vi "writePre.vi"(1 "input_data":u8[](array[numeric]) format="%.0x", 2 "address":u8, 3 "Channel":u8 max=5 step=1, 4 "order":u8[](array[numeric])=[238, 0, 13, 0, 1, 160, 0, 0, 169, 255, 252, 255, 255] format="%.0x") -> (0 "out":u8[](array[numeric]) format="%.0x")   [LabVIEW 2011]
panel:
  out "输出数组":u8[](array[numeric]) format="%.0x"
  out "size":u8
  # "channel"
  # "芯片地址"
  # "写入字节数"
  # "读写控制"
  # "字节数"
  # "写入地址"
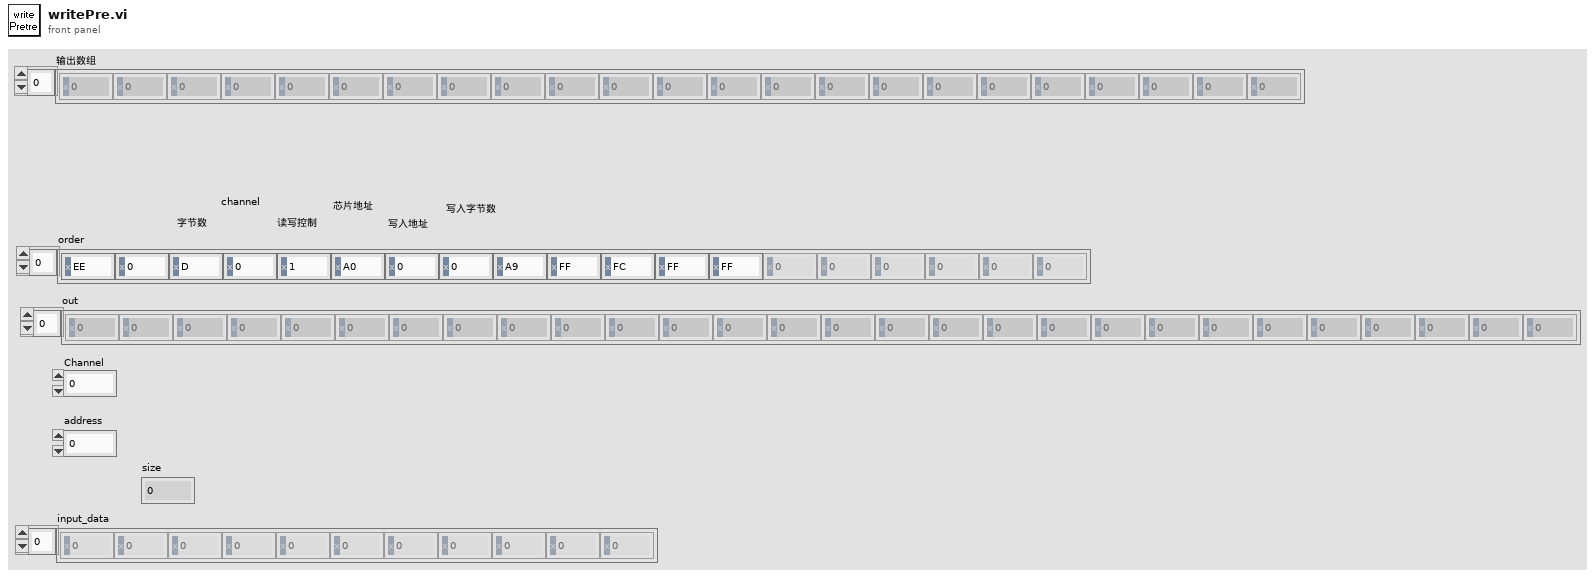
[diagram p1: front panel]
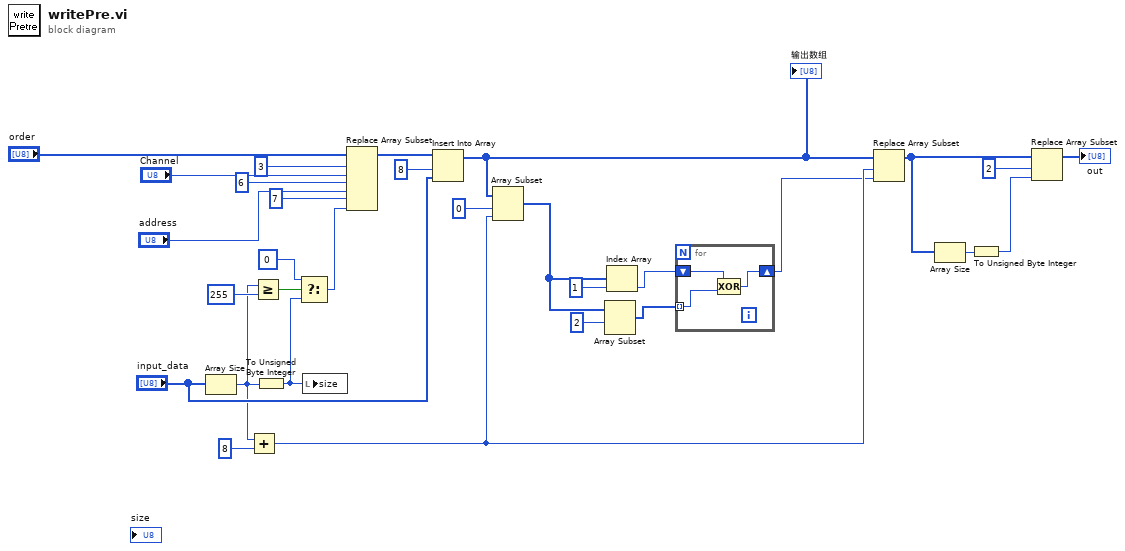
[diagram p0: block diagram]
diagram:
  n1 = Array Size(array="input_data") -> (size(s)=w3:i32)
  n2 = Add(x=w3, y=8) -> (x+y=w13:i32)
  n3 = Greater Or Equal?(x=w3, y=255) -> (x >= y?=w5:bool)
  n4 = To Unsigned Byte Integer(number=w3) -> (unsigned 8bit integer=w1:u8)
  n5 = Select(t=u8 0, s=w5, f=w1) -> (s? t:f=w2:u8)
  n6 = local write "size"(w1) -> ()
  n7 = Replace Array Subset(array="order", new element #1="Channel", index #1=3 ("索引"), new element #2="address", index #2=6 ("索引"), new element #3=w2, index #3=7 ("索引")) -> (w24:u8[])
  n8 = Insert Into Array(array=w24, index=8 ("索引"), new element="input_data") -> (w14:u8[])
  "输出数组" <- w14
  n9 = Array Subset(array=w14, index=0 ("索引"), length=w13) -> (w15:u8[])
  n10 = Array Subset(array=w15, index=2 ("索引")) -> (w16:u8[])  [unwired: 1 in]
  n11 = Index Array(array=w15, index=1 ("索引")) -> (element=w17:u8)
  n12 = for {
    shift-right: [w31] -> w12
    shift-left: w17 -> [w33]
    tunnel: w16 -> [w32] mode=indexing
    n13 = Compound Arithmetic op=XOR(w33, w32) -> (w31:u8)
  }
  n14 = Replace Array Subset(array=w14, new element=w12, index=w13) -> (w10:u8[])
  n15 = Array Size(array=w10) -> (size(s)=w11:i32)
  n16 = To Unsigned Byte Integer(number=w11) -> (unsigned 8bit integer=w9:u8)
  n17 = Replace Array Subset(array=w10, new element=w9, index=2 ("索引")) -> (→"out":u8[])
